vi "get boat location.vi"(2 "Tug":string="L", 3 "Nav String":string="$,G,43,13,230,P,10,20,120,T,10,10,330,L,14,36,110,A,3,5,B,7,8,C,16,20,D,-1,-1,S,08,12,234\r") -> (0 "Valid ?":bool)   [LabVIEW 2013]
doc: "This VI gets the location for the Tug specified along with the time data for the data. The output cluster has which boat it is, x, y, and angle, in that order."
panel:
  out "Nav Data":T1
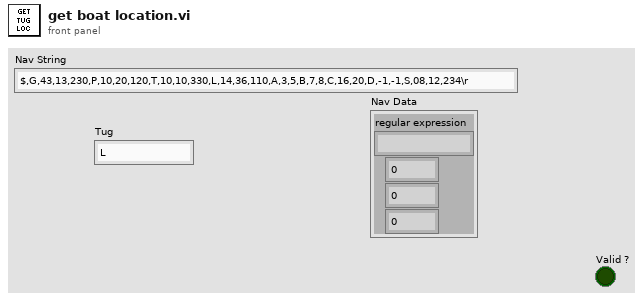
[diagram p1: front panel]
types:
  T1 = cluster{"regular expression":string, i32, i32, i32}
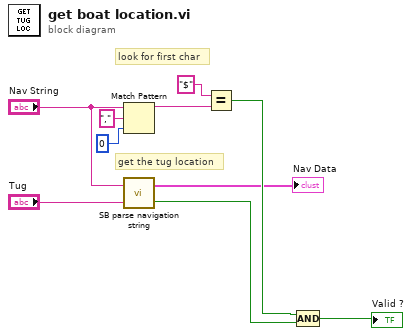
[diagram p0: block diagram]
diagram:
  # "get the tug location"
  # "look for first char"
  n1 = Match Pattern(string="Nav String", regular expression=",", offset (0)=0) -> (before substring=w9:string)  [unwired: 3 out]
  n2 = call "SB parse navigation string.vi"("Header"="Tug", "Nav String"="Nav String") -> ("Valid?"=w4:bool, "Nav Data"=→"Nav Data":T1)
  n3 = Equal?(x="$", y=w9) -> (x = y?=w5:bool)
  n4 = Compound Arithmetic op=AND(w5, w4) -> (→"Valid ?":bool)
